vi "DiscoveryService UnregisterService.vi"(8 "error in":errorcluster, 9 "timeout (ms)":i32=-1, 10 "Request Data":T2, 11 "gRPC ID":T3) -> (0 "error out":errorcluster, 2 "Response Data":T1, 3 "gRPC ID out":T3)   [LabVIEW 2020, in "Discovery_client.lvlib"]
uses:
  Discovery_client.lvlib
  <vilib>/gRPC/LabVIEW gRPC Library/Shared/grpcId.ctl
  RPC Messages/ni_measurementlink_discovery_v1_UnregisterServiceRequest.ctl
  RPC Messages/ni_measurementlink_discovery_v1_UnregisterServiceResponse.ctl
  3477ff3c-ac1a-41b2-98e0-1f89dff8fa77.vi
  <vilib>/gRPC/LabVIEW gRPC Library/Shared/TranslateGrpcError.vi
  <vilib>/gRPC/LabVIEW gRPC Library/Shared/Wait On Occurence.vi
  <vilib>/AdvancedString/1D String Array to Delimited String.vi
  <vilib>/gRPC/LabVIEW gRPC Library/Server API/Server/Get Server DLL Path.vi
  <vilib>/gRPC/LabVIEW gRPC Library/grpc-lvsupport-release.lvlib
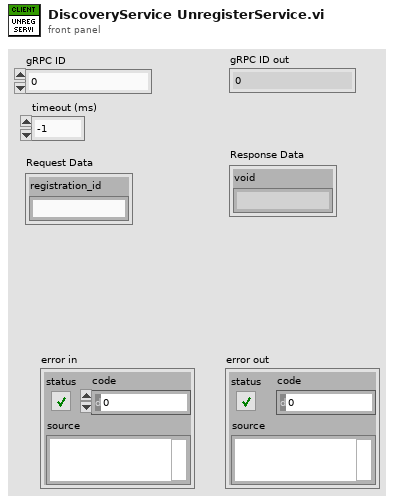
[diagram p1: front panel]
types:
  T1 = typedef "Discovery_client.lvlib/ni_measurementlink_discovery_v1_UnregisterServiceResponse.ctl" = cluster{"void":string}
  T2 = typedef "Discovery_client.lvlib/ni_measurementlink_discovery_v1_UnregisterServiceRequest.ctl" = cluster{"registration_id":string}
  T3 = typedef "grpc-lvsupport-release.lvlib/grpcId.ctl" = u64
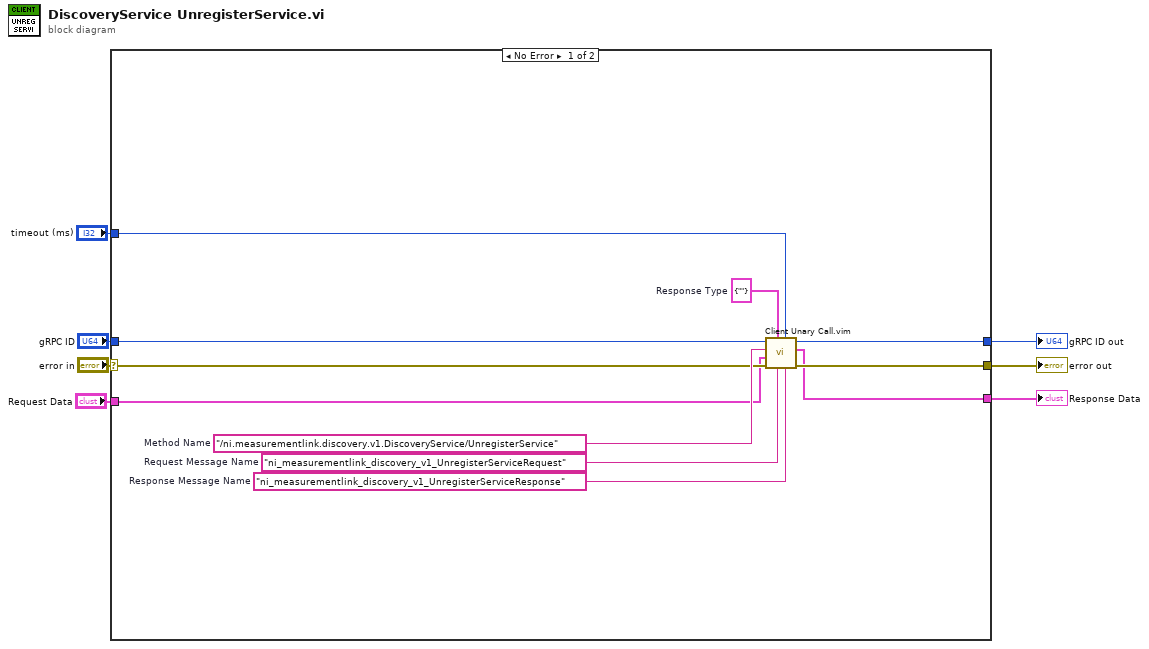
[diagram p0: block diagram]
diagram:
  n1 = case shown="No Error" "error in" {
    selector: "error in" -> [w14 w19]
    tunnel: [w13 w19] -> w6
    tunnel: "gRPC ID" -> [w12 w20]
    tunnel: [w11 w20] -> w4
    tunnel: "Request Data" -> [w10 _]
    tunnel: [w9 _] -> w2
    tunnel: "timeout (ms)" -> [w8 _]
    frame No Error {
      w15 = "ni_measurementlink_discovery_v1_UnregisterServiceResponse"  # Response Message Name
      w16 = "ni_measurementlink_discovery_v1_UnregisterServiceRequest"  # Request Message Name
      w17 = T1 {"void"=""}  # Response Type
      w18 = "/ni.measurementlink.discovery.v1.DiscoveryService/UnregisterService"  # Method Name
      n2 = call "Client Unary Call.vim"("Response Message Name"=w15, "timeout (ms)"=w8, "Request Message Name"=w16, "Response Type"=w17, "error in"=w14, "Request Data"=w10, "Method Name"=w18, "ClientID in"=w12) -> ("error out"=w13:errorcluster, "Response Data"=w9:T1, "ClientID out"=w11:u64)  [unwired: 1 in]
    }
    frame Error {
    }
  }
  "error out" <- w6
  "gRPC ID out" <- w4
  "Response Data" <- w2
